vi "Example_scope.vi"() -> ()   [LabVIEW 2012, in "AnalogDiscSDKLv.lvlib"]
uses:
  <instrlib>/AnalogDiscSDKLv/AnalogDiscSDKLv.lvlib
  <instrlib>/AnalogDiscSDKLv/VIs/DWF_AcqMode.ctl
  <instrlib>/AnalogDiscSDKLv/VIs/DWF_TrigSrc.ctl
  <instrlib>/AnalogDiscSDKLv/VIs/DWF_Filter.ctl
  <instrlib>/AnalogDiscSDKLv/VIs/DWF_InstrumentStatus.ctl
  Windows/System32/dwf.dll
panel:
  out "src":i32
  out "pfstrigsrc 2":i32
  out "pfstrigsrc":i32 format="%b"
  in  "secTimeout":dbl
  out "rate":sgl
  in  "Quit":bool
  out "Array":T1[](array[typedef])
  out "psts":T1
  out "initialized array":dbl[](array[numeric])
  out "Waiting Counter":i32
  out "function return 7":i32
  out "size(s) 2":i32
  out "size(s)":i32
  out "rgdSamples out":dbl[](graph)
  out "hdwf":i32
  out "DeviceID":i32[](array[numeric])
  out "UserName":string
  out "SN":string
  out "DevName":string
  out "pnDevice":i32
  out "isBusy":i32[](array[numeric])
  out "DeviceVersion":i32[](array[numeric])
  out "function return 6":i32
  out "function return 5":i32
  out "function return 4":i32
  out "function return 3":i32
  out "function return 2":i32
  in  "indexCh":i32
  in  "Enable":i32=1
  in  "Filter":T2
  in  "trigsrc":T3
  in  "voltOffset":dbl
  in  "voltsRange":dbl=5.0
  in  "nSize":i32=1024
  in  "hzFrquency":dbl=100000000.0 format="%#_6p"
  in  "AcqMode":T4
  in  "fStart":i32=1
  in  "fReconfigure":i32
  in  "fAutoConfig":i32=1
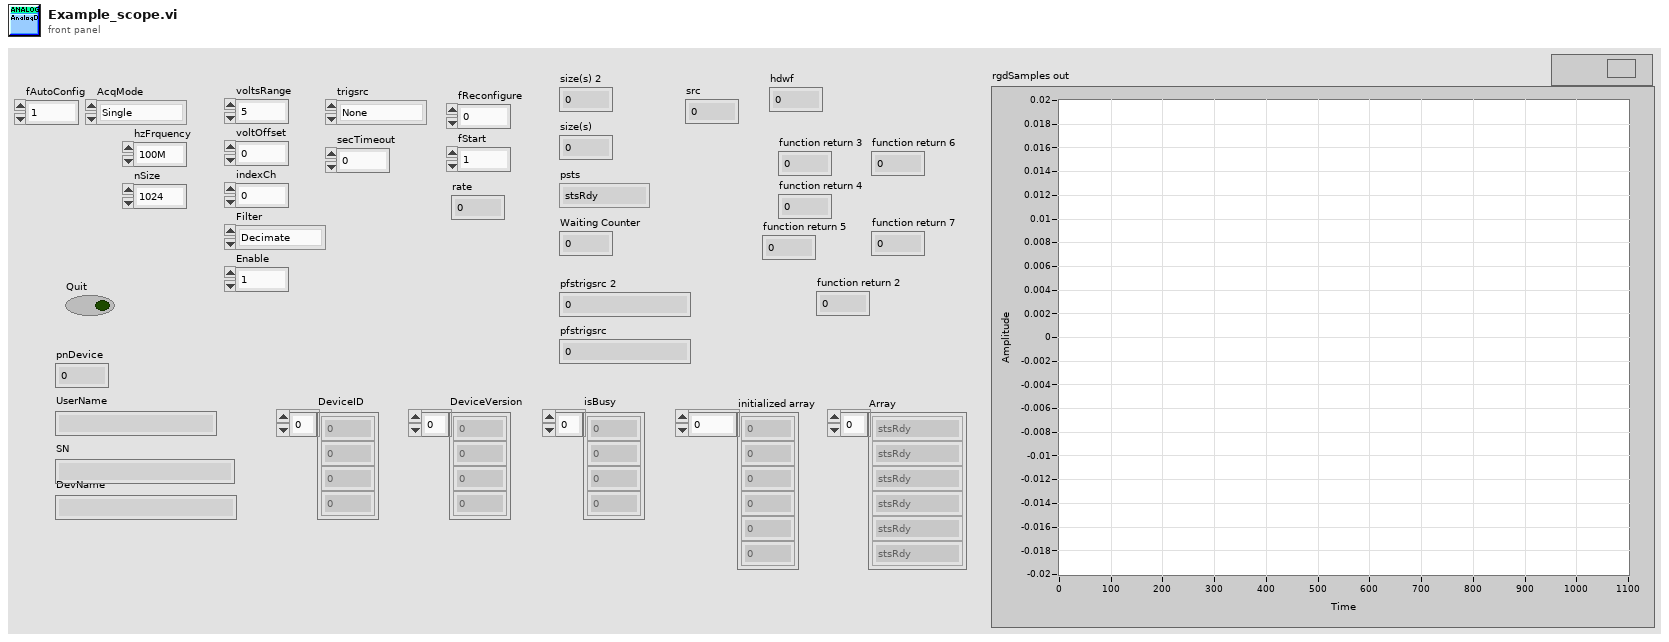
[diagram p1: front panel]
types:
  T1 = typedef "DWF_InstrumentStatus.ctl" = enum16{"stsRdy", "stsARM", "stsDone", "stsTrig", "stsCfg", "stsPrefill", "stsNotDone", "stsTrigDly", "stsError", "stsBusy", "stsStop"}
  T2 = typedef "DWF_Filter.ctl" = enum16{"Decimate", "Average", "MinMax"}
  T3 = typedef "DWF_TrigSrc.ctl" = enum16{"None", "PC", "DetectorAnalogIn", "DetectorDigitalIn", "AnalogIn", "DigitalIn", "DigitalOut", "AnalogOut1", "AnalogOut2", "AnalogOut3", "AnalogOut4", "External1", "External2", "External3", "External4"}
  T4 = typedef "DWF_AcqMode.ctl" = enum16{"Single", "ScanShift", "ScanScreen", "Record"}
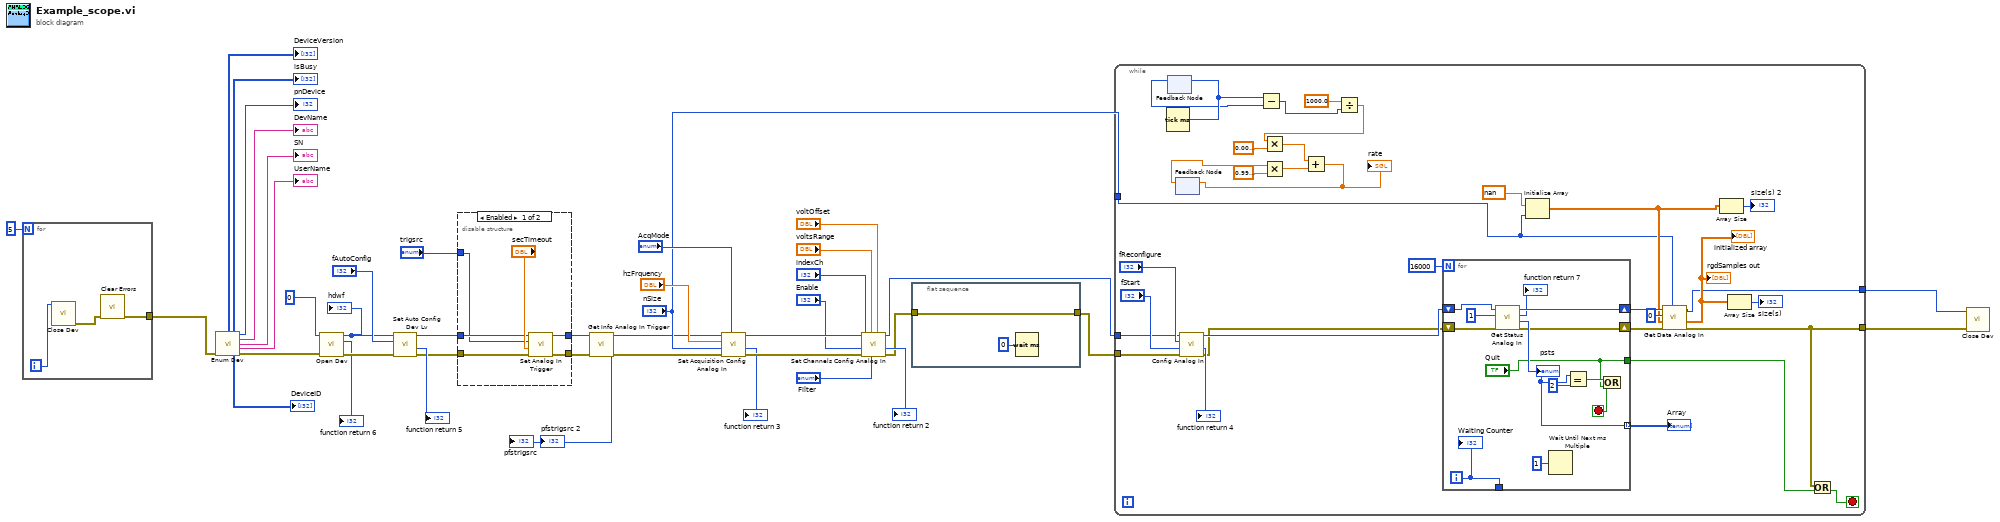
[diagram p0: block diagram]
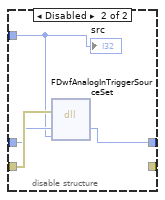
[diagram p2: hidden frame]
diagram:
  n1 = for {
    N: 5 -> [_]
    tunnel: [w42] -> w13
    i -> [w43]
    n2 = call <instrlib>:"Close Dev.vi"("hdwf"=w43) -> ("error out"=w44:errorcluster)  [unwired: 9 in, 1 out]
    n3 = call <vilib>:"Clear Errors.vi"("error in (no error)"=w44) -> ("error out"=w42:errorcluster)  [unwired: 6 in]
  }
  n4 = call <instrlib>:"Enum Dev.vi"("error in (no error)"=w13) -> ("DeviceVersion"=→"DeviceVersion":i32[], "isBusy"=→"isBusy":i32[], "pnDevice"=→"pnDevice":i32, "DevName"=→"DevName":string, "SN"=→"SN":string, "UserName"=→"UserName":string, "DeviceID"=→"DeviceID":i32[], "error out"=w25:errorcluster)  [unwired: 6 in, 1 out]
  n5 = call <instrlib>:"Open Dev.vi"("error in (no error)"=w25, "idxDev"=0) -> ("error out"=w39:errorcluster, "function return"=→"function return 6":i32, "hdwf"=w40:i32)  [unwired: 7 in]
  "hdwf" <- w40
  n6 = call <instrlib>:"Set Auto Config Dev Lv.vi"("error in (no error)"=w39, "fAutoConfig"="fAutoConfig", "hdwf"=w40) -> ("error out"=w6:errorcluster, "function return"=→"function return 5":i32, "hdwf out"=w7:i32)  [unwired: 6 in]
  n7 = disable-structure shown="Enabled" {
    disable-tunnel: [w49 w52] -> w11
    disable-tunnel: w7 -> [w48 w53]
    disable-tunnel: w6 -> [w47 w54]
    disable-tunnel: [w46 _] -> w5
    disable-tunnel: "trigsrc" -> [w45 w51]
    frame Enabled {
      n8 = call <instrlib>:"Set Analog In Trigger.vi"("error in (no error)"=w47, "timeout"="secTimeout", "trigsrc"=w45, "hdwf"=w48) -> ("error out"=w46:errorcluster, "hdwf out"=w49:i32)  [unwired: 6 in]
    }
    frame Disabled {
      n9 = dll-call lib="C:/Windows/System32/dwf.dll" fn="FDwfAnalogInTriggerSourceSet"(error in=w54, "hdwf"=w53, "trigsrc"=w51) -> ("hdwf"=w52:i32)  [unwired: 4 in, 2 out]
      "src" <- w51
    }
  }
  n10 = call <instrlib>:"Get Info Analog In Trigger.vi"("error in (no error)"=w5, "hdwf"=w11) -> ("error out"=w4:errorcluster, "pfstrigsrc"=→"pfstrigsrc":i32, "hdwf out"=w8:i32)  [unwired: 7 in]
  n11 = call <instrlib>:"Set Acquisition Config Analog In.vi"("AcqMode"="AcqMode", "error in (no error)"=w4, "nSize"="nSize", "hzFrquency"="hzFrquency", "hdwf"=w8) -> ("error out"=w38:errorcluster, "function return"=→"function return 3":i32, "hdwf out"=w37:i32)  [unwired: 4 in]
  n12 = call <instrlib>:"Set Channels Config Analog In.vi"("voltOffset"="voltOffset", "Filter"="Filter", "voltsRange"="voltsRange", "error in (no error)"=w38, "Enable"="Enable", "indexCh"="indexCh", "hdwf"=w37) -> ("error out"=w9:errorcluster, "function return"=→"function return 2":i32, "hdwf out"=w3:i32)  [unwired: 2 in]
  n13 = flat-sequence {
    tunnel: w9 -> [w55]
    tunnel: [w55] -> w12
    frame #0 {
      n14 = Wait (ms)(milliseconds to wait=u32 0) -> ()  [unwired: 1 out]
    }
  }
  n15 = while {
    tunnel: w12 -> [w86]
    tunnel: w3 -> [w85]
    tunnel: [w71] -> w24
    tunnel: "nSize" -> [w75]
    tunnel: [w70] -> w15
    stop <- w72 stop-if-true
    n16 = Tick Count (ms)() -> (millisecond timer value=w63:u32)
    n17 = feedback-in #1(w63) -> ()
    n18 = feedback #1() -> (w62:u32)  [unwired: 1 in]
    n19 = feedback #2() -> (w67:dbl)  [unwired: 1 in]
    n20 = call <instrlib>:"Config Analog In.vi"("error in (no error)"=w86, "fStart"="fStart", "fReconfigure"="fReconfigure", "hdwf"=w85) -> ("error out"=w58:errorcluster, "function return"=→"function return 4":i32, "hdwf out"=w84:i32)  [unwired: 5 in]
    n21 = Subtract(x=w63, y=w62) -> (x-y=w60:u32)
    n22 = Multiply(x=w67, y=sgl 0.99) -> (x*y=w68:dbl)
    n23 = Divide(x=1000.0, y=w60) -> (x/y=w59:dbl)
    n24 = Multiply(x=w59, y=sgl 0.01) -> (x*y=w69:dbl)
    n25 = Add(x=w69, y=w68) -> (x+y=w66:dbl)
    "rate" <- w66
    n26 = feedback-in #2(w66) -> ()
    n27 = for {
      N: 16000 -> [_]
      shift-right: [w101] -> w83
      shift-left: w84 -> [w102]
      shift-right: [w91] -> w82
      shift-left: w58 -> [w99]
      tunnel: [w93] -> _
      tunnel: [w95] -> w74 mode=indexing
      tunnel: ["Quit"] -> w57
      i -> [w93]
      stop <- w92 stop-if-true
      n28 = call <instrlib>:"Get Status Analog In.vi"("error in (no error)"=w99, "fReadData"=1, "hdwf"=w102) -> ("error out"=w91:errorcluster, "psts"=w95:T1, "function return"=→"function return 7":i32, "hdwf out"=w101:i32)  [unwired: 4 in]
      "psts" <- w95
      n29 = Wait Until Next ms Multiple(millisecond multiple=u32 1) -> ()  [unwired: 1 out]
      n30 = Equal?(x=w95, y=u8 2) -> (x = y?=w96:bool)
      n31 = Or(x=w96, y="Quit") -> (x .or. y?=w92:bool)
      "Waiting Counter" <- w93
    }
    "Array" <- w74
    n32 = Initialize Array(nan ("Numeric"), w75) -> (w77:dbl[])
    n33 = call <instrlib>:"Get Data Analog In.vi"("BufferSize"=w75, "error in (no error)"=w82, "rgdSamples"=w77, "idxChannel"=0, "hdwf"=w83) -> ("error out"=w71:errorcluster, "rgdSamples out"=w76:dbl[], "function return"=w70:i32)  [unwired: 4 in]
    "rgdSamples out" <- w76
    "initialized array" <- w76
    n34 = Array Size(array=w77) -> (size(s)=→"size(s) 2":i32)
    n35 = Array Size(array=w76) -> (size(s)=→"size(s)":i32)
    n36 = Or(x=w71, y=w57) -> (x .or. y?=w72:bool)
  }
  n37 = call <instrlib>:"Close Dev.vi"("error in (no error)"=w24, "hdwf"=w15) -> ()  [unwired: 8 in, 2 out]
